vi "Offset_Error&Warnings.vi"(1 "Cluster":T1) -> ()   [LabVIEW 2011]
panel:
  out "String":string
  out "DEC off":dbl format="%.2g"
  out "RA off":dbl format="%.2g"
  out "Warning Code":u8
  out "Error Code":u8
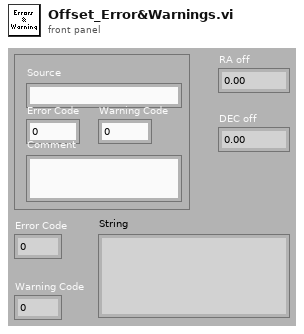
[diagram p1: front panel]
types:
  T1 = cluster{"Source":string, "Error Code":u32, "Warning Code":u32, "Comment":string}
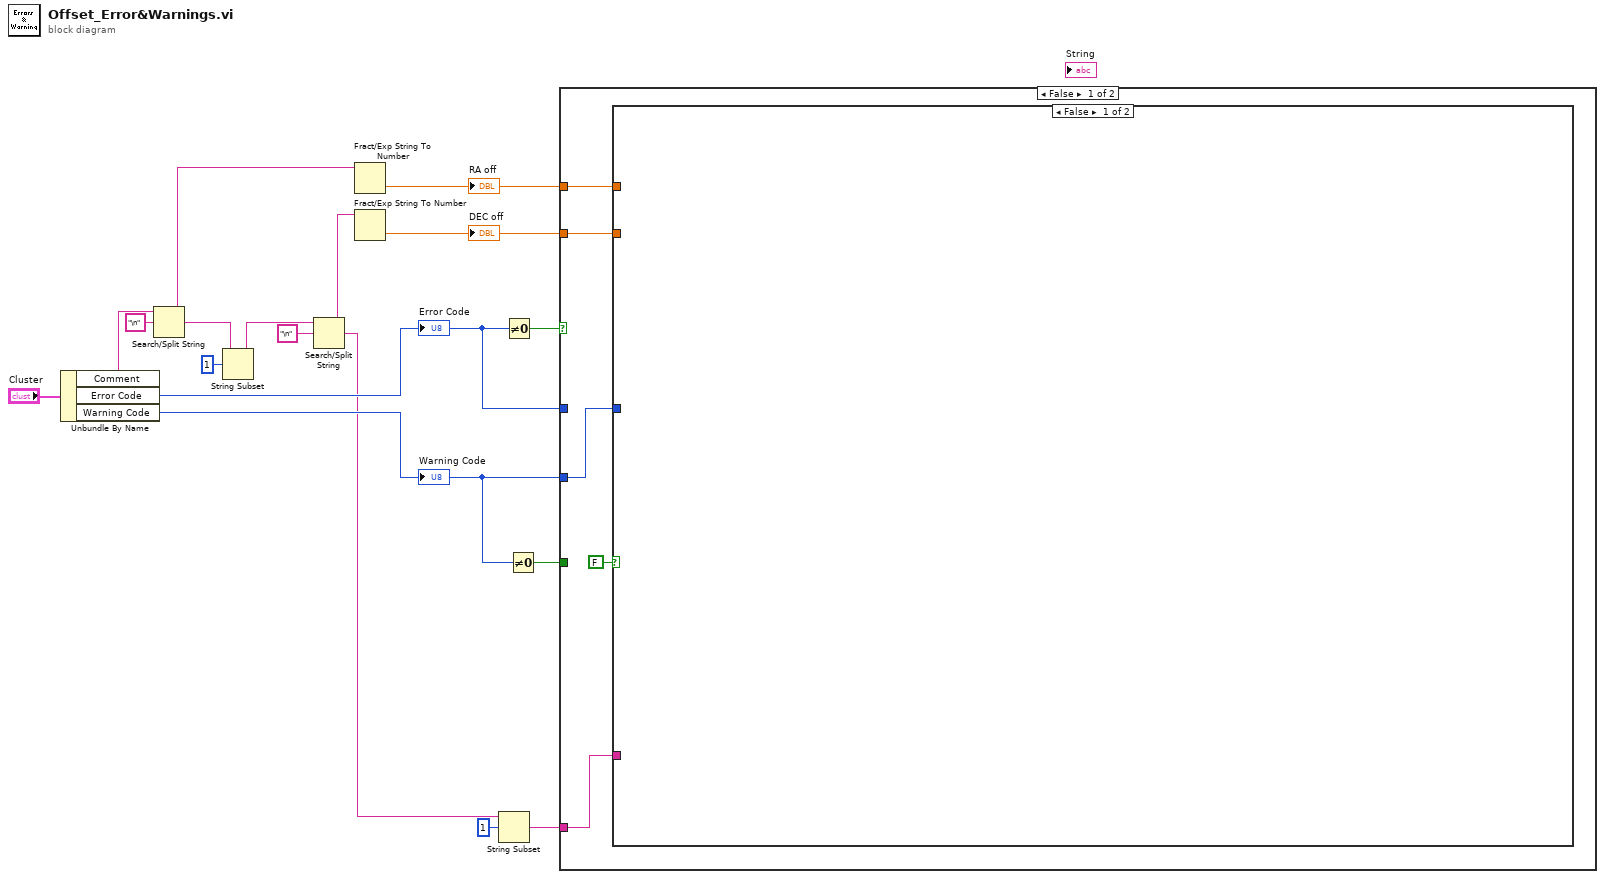
[diagram p0: block diagram]
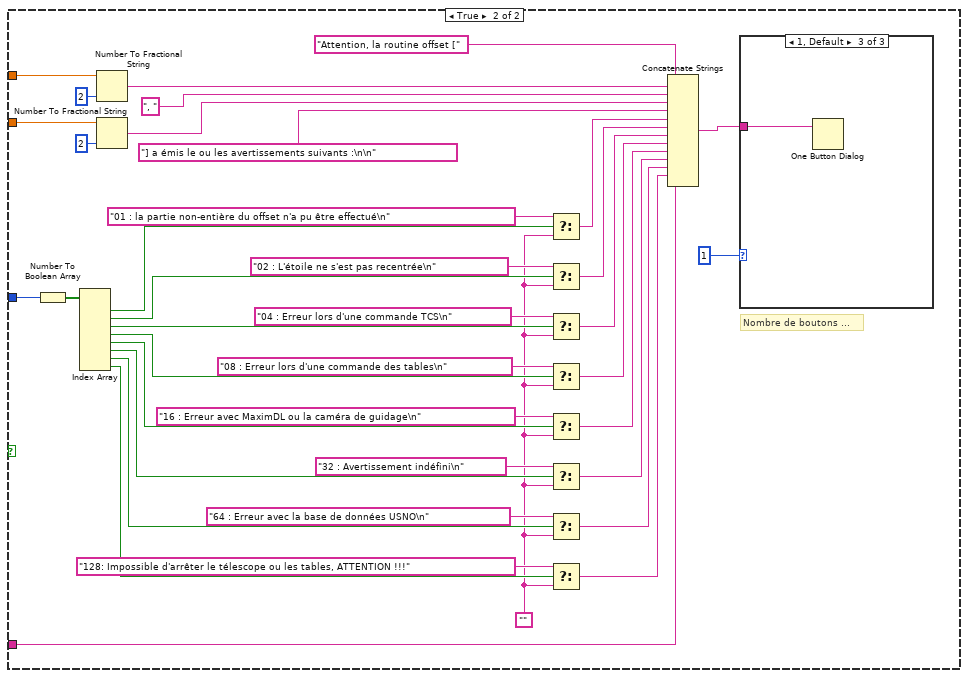
[diagram p2: hidden frame]
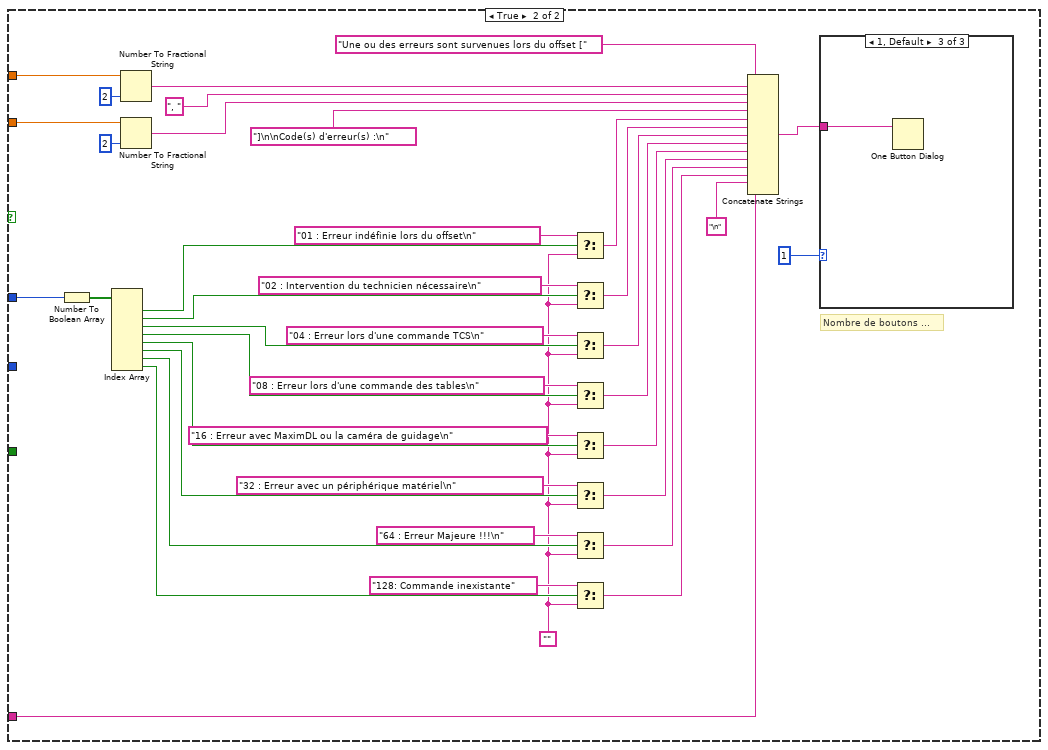
[diagram p5: hidden frame]
diagram:
  n1 = Unbundle By Name("Cluster") -> ("Comment"=w13:string, "Error Code"=w15:u32, "Warning Code"=w14:u32)
  "Error Code" <- w15
  "Warning Code" <- w14
  n2 = Search/Split String(string=w13, search string/char (-)="\n") -> (substring before match=w8:string, match + rest of string=w2:string)  [unwired: 1 in, 1 out]
  n3 = String Subset(string=w2, offset (0)=1) -> (substring=w1:string)  [unwired: 1 in]
  n4 = Search/Split String(string=w1, search string/char (-)="\n") -> (substring before match=w7:string, match + rest of string=w5:string)  [unwired: 1 in, 1 out]
  n5 = Fract/Exp String To Number(string=w8) -> (number=w10:dbl)  [unwired: 3 in, 1 out]
  "RA off" <- w10
  n6 = Fract/Exp String To Number(string=w7) -> (number=w9:dbl)  [unwired: 3 in, 1 out]
  "DEC off" <- w9
  n7 = String Subset(string=w5, offset (0)=1) -> (substring=w6:string)  [unwired: 1 in]
  n8 = Not Equal To 0?(x=w15) -> (x != 0?=w18:bool)
  n9 = Not Equal To 0?(x=w14) -> (x != 0?=w17:bool)
  n10 = case shown="False" w18 {
    tunnel: w15 -> [_ w92]
    tunnel: w14 -> [w21 _]
    tunnel: w10 -> [w23 w101]
    tunnel: w9 -> [w22 w100]
    tunnel: w17 -> [_ _]
    tunnel: w6 -> [w20 w65]
    frame False {
      n11 = case shown="False" FALSE {
        tunnel: w23 -> [_ w27]
        tunnel: w22 -> [_ w26]
        tunnel: w21 -> [_ w25]
        tunnel: w20 -> [_ w24]
        frame False {
        }
        frame True {
          w36 = ""
          # "Nombre de boutons ..."
          n12 = Number To Boolean Array(number=w25) -> (Boolean array=w53:bool[])
          n13 = Index Array(array=w53) -> (element #1=w52:bool, element #2=w51:bool, element #3=w50:bool, element #4=w49:bool, element #5=w48:bool, element #6=w47:bool, element #7=w46:bool, element #8=w45:bool)  [unwired: 8 in]
          n14 = Number To Fractional String(number=w27, precision (6)=i16 2) -> (F-format string=w59:string)  [unwired: 2 in]
          n15 = Number To Fractional String(number=w26, precision (6)=i16 2) -> (F-format string=w57:string)  [unwired: 2 in]
          n16 = Select(t="01 : la partie non-entière du offset n'a pu être effectué\n", s=w52, f=w36) -> (s? t:f=w35:string)
          n17 = Select(t="02 : L'étoile ne s'est pas recentrée\n", s=w51, f=w36) -> (s? t:f=w34:string)
          n18 = Select(t="04 : Erreur lors d'une commande TCS\n", s=w50, f=w36) -> (s? t:f=w33:string)
          n19 = Select(t="08 : Erreur lors d'une commande des tables\n", s=w49, f=w36) -> (s? t:f=w32:string)
          n20 = Select(t="16 : Erreur avec MaximDL ou la caméra de guidage\n", s=w48, f=w36) -> (s? t:f=w31:string)
          n21 = Select(t="32 : Avertissement indéfini\n", s=w47, f=w36) -> (s? t:f=w30:string)
          n22 = Select(t="64 : Erreur avec la base de données USNO\n", s=w46, f=w36) -> (s? t:f=w29:string)
          n23 = Select(t="128: Impossible d'arrêter le télescope ou les tables, ATTENTION !!!", s=w45, f=w36) -> (s? t:f=w28:string)
          n24 = Concatenate Strings("Attention, la routine offset [", w59, ", ", w57, "] a émis le ou les avertissements suivants :\n\n", w35, w34, w33, w32, w31, w30, w29, w28, w24) -> (w55:string)
          n25 = case shown="1, Default" 1 {
            tunnel: w55 -> [_ _ w63]
            frame 2 {
            }
            frame 3 {
            }
            frame 1, Default {
              n26 = One Button Dialog(message=w63) -> ()  [unwired: 1 in, 1 out]
            }
          }
        }
      }
    }
    frame True {
      w74 = ""
      # "Nombre de boutons ..."
      n27 = Number To Boolean Array(number=w92) -> (Boolean array=w91:bool[])
      n28 = Index Array(array=w91) -> (element #1=w90:bool, element #2=w89:bool, element #3=w88:bool, element #4=w87:bool, element #5=w86:bool, element #6=w85:bool, element #7=w84:bool, element #8=w83:bool)  [unwired: 8 in]
      n29 = Number To Fractional String(number=w101, precision (6)=i16 2) -> (F-format string=w98:string)  [unwired: 2 in]
      n30 = Number To Fractional String(number=w100, precision (6)=i16 2) -> (F-format string=w96:string)  [unwired: 2 in]
      n31 = Select(t="01 : Erreur indéfinie lors du offset\n", s=w90, f=w74) -> (s? t:f=w73:string)
      n32 = Select(t="02 : Intervention du technicien nécessaire\n", s=w89, f=w74) -> (s? t:f=w72:string)
      n33 = Select(t="04 : Erreur lors d'une commande TCS\n", s=w88, f=w74) -> (s? t:f=w71:string)
      n34 = Select(t="08 : Erreur lors d'une commande des tables\n", s=w87, f=w74) -> (s? t:f=w70:string)
      n35 = Select(t="16 : Erreur avec MaximDL ou la caméra de guidage\n", s=w86, f=w74) -> (s? t:f=w69:string)
      n36 = Select(t="32 : Erreur avec un périphérique matériel\n", s=w85, f=w74) -> (s? t:f=w68:string)
      n37 = Select(t="64 : Erreur Majeure !!!\n", s=w84, f=w74) -> (s? t:f=w67:string)
      n38 = Select(t="128: Commande inexistante", s=w83, f=w74) -> (s? t:f=w66:string)
      n39 = Concatenate Strings("Une ou des erreurs sont survenues lors du offset [", w98, ", ", w96, "]\n\nCode(s) d'erreur(s) :\n", w73, w72, w71, w70, w69, w68, w67, w66, "\n" ("string"), w65) -> (w94:string)
      n40 = case shown="1, Default" 1 {
        tunnel: w94 -> [_ _ w104]
        frame 2 {
        }
        frame 3 {
        }
        frame 1, Default {
          n41 = One Button Dialog(message=w104) -> ()  [unwired: 1 in, 1 out]
        }
      }
    }
  }
